vi "get_distance.vi"(8 "error in (no error)":errorcluster, 11 "TrajectoryDL110420DoubleCircle in":refnum<class "TrajectoryDL110420DoubleCircle.lvclass">) -> (0 "error out":errorcluster, 2 "distance":dbl[unit], 3 "TrajectoryDL110420DoubleCircle out":refnum<class "TrajectoryDL110420DoubleCircle.lvclass">)   [LabVIEW 2010, in "TrajectoryDL110420DoubleCircle.lvclass"]
uses:
  TrajectoryDL110420DoubleCircle.lvclass
  common/classes/SpaceVector/SpaceVector/SpaceVector.lvclass
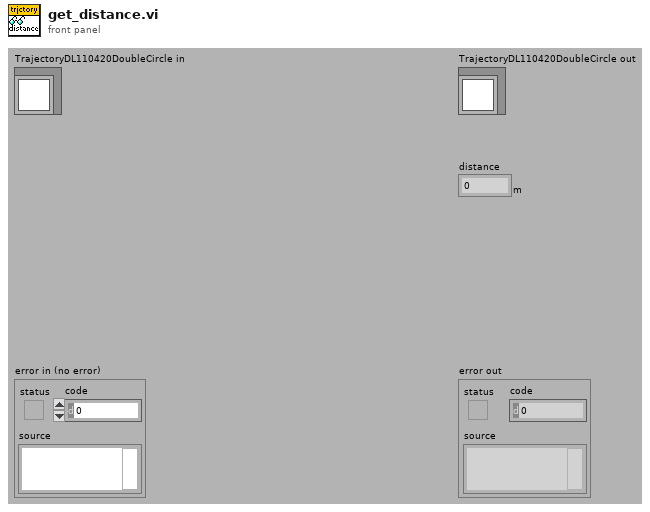
[diagram p1: front panel]
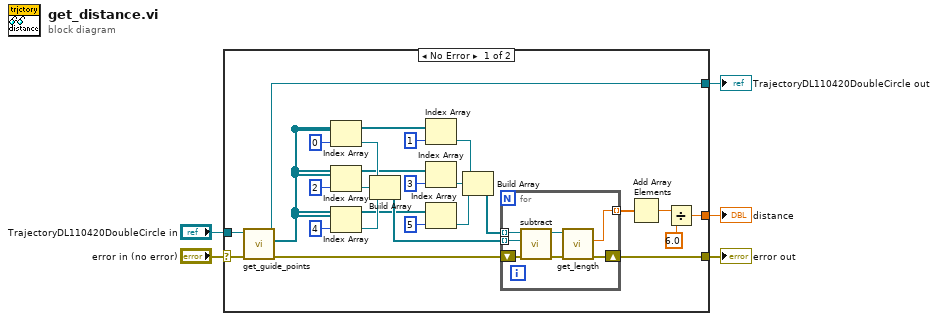
[diagram p0: block diagram]
diagram:
  n1 = case shown="No Error" "error in (no error)" {
    selector: "error in (no error)" -> [w9 w38]
    tunnel: [w20 w38] -> w4
    tunnel: [w6 w37] -> w2
    tunnel: "TrajectoryDL110420DoubleCircle in" -> [w7 w37]
    tunnel: [w19 _] -> w1
    frame No Error {
      n2 = call-dynamic "get_guide_points.vi"("error in (no error)"=w9, "TrajectoryDL110420DoubleCircle in"=w7) -> ("error out"=w8:errorcluster, "guide points"=w10:refnum<class "SpaceVector.lvclass">[], "TrajectoryDL110420DoubleCircle out"=w6:refnum<class "TrajectoryDL110420DoubleCircle.lvclass">)  [unwired: 7 in]
      n3 = Index Array(array=w10, index=0) -> (element=w18:refnum<class "SpaceVector.lvclass">)
      n4 = Index Array(array=w10, index=2) -> (element=w17:refnum<class "SpaceVector.lvclass">)
      n5 = Index Array(array=w10, index=4) -> (element=w16:refnum<class "SpaceVector.lvclass">)
      n6 = Build Array(w18, w17, w16) -> (w11:refnum<class "SpaceVector.lvclass">[])
      n7 = Index Array(array=w10, index=1) -> (element=w15:refnum<class "SpaceVector.lvclass">)
      n8 = Index Array(array=w10, index=3) -> (element=w14:refnum<class "SpaceVector.lvclass">)
      n9 = Index Array(array=w10, index=5) -> (element=w13:refnum<class "SpaceVector.lvclass">)
      n10 = Build Array(w15, w14, w13) -> (w12:refnum<class "SpaceVector.lvclass">[])
      n11 = for {
        shift-right: [w34] -> w20
        shift-left: w8 -> [w33]
        tunnel: [w32] -> w23 mode=indexing
        tunnel: w12 -> [w31] mode=indexing
        tunnel: w11 -> [w30] mode=indexing
        n12 = call "subtract.vi"("error in (no error)"=w33, "subtrahend"=w30, "SpaceVector in"=w31) -> ("error out"=w36:errorcluster, "SpaceVector out"=w35:refnum<class "SpaceVector.lvclass">)  [unwired: 7 in]
        n13 = call "get_length.vi"("error in (no error)"=w36, "SpaceVector in"=w35) -> ("error out"=w34:errorcluster, "length"=w32:dbl[unit])  [unwired: 7 in, 1 out]
      }
      n14 = Add Array Elements(numeric array=w23) -> (sum=w22:dbl[unit])
      n15 = Divide(x=w22, y=6.0) -> (x/y=w19:dbl[unit])
    }
    frame Error {
    }
  }
  "error out" <- w4
  "TrajectoryDL110420DoubleCircle out" <- w2
  "distance" <- w1
